vi "Heater PSU server.vi"() -> ()   [LabVIEW 2024]
doc: "Vi provides top level control program for TTICPX200 PSU used to drive the motor heater in the mechanical LTM"
uses:
  <userlib>/_OpenG.lib/comparison/comparison.llb/Boolean Changed__ogtk.vi
  <userlib>/_OpenG.lib/comparison/comparison.llb/DBL Changed__ogtk.vi
  <instrlib>/TTI CPX400/TTI CPX400.lvlib
  <userlib>/_OpenG.lib/comparison/comparison.llb/openg_comparison__ogtk.lvlib
panel:
  in  "Current Limit (600mA)":dbl=0.6 format="%.2g"
  out "Heater Monitor":waveform(dbl)[](array[waveform])
  in  "Heater PSU \nVISA name":refnum<visa-resource-name>="CPX400PSU"
  in  "Cadence":i64=100 min=1 max=1000
  out "Voltage":waveform(dbl)={"t0"=timestamp(3819958139.6161337 s since 1904-01-01), "dt"=1.0, "Y"=[-0.006], "attributes"=variant("NI_ChannelName"=variant(string "Heater_Voltage"))}
  out "I&V (Graph)":dynamicdata(graph)=[{"t0"=timestamp(3819958139.6161337 s since 1904-01-01), "dt"=1.0, "Y"=[-0.006], "attributes"=variant("NI_ChannelName"=variant(string "Heater_Voltage"))}, {"t0"=timestamp(3819958139.6161337 s since 1904-01-01), "dt"=1.0, "Y"=[-0.002], "attributes"=variant("NI_ChannelName"=variant(string "Heater_Current"))}]
  out "Current":waveform(dbl)={"t0"=timestamp(3819958139.6161337 s since 1904-01-01), "dt"=1.0, "Y"=[-0.002], "attributes"=variant("NI_ChannelName"=variant(string "Heater_Current"))}
  in  "stop":bool
  in  "Enable Output (T: Enable)":bool
  in  "Set Voltage":dbl=0.92 min=0.0 max=1.0 step=0.01 format="%.2f"
  in  "OCP Current (A)":dbl=1.0
  in  "OVP Voltage (V)":dbl=1.0
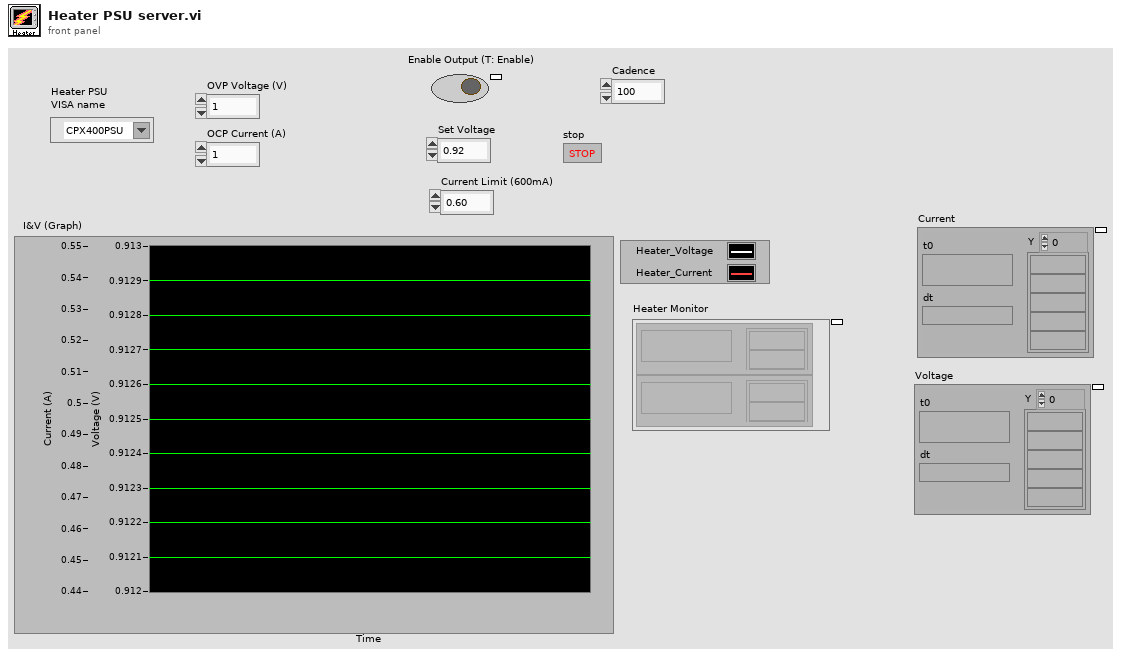
[diagram p1: front panel]
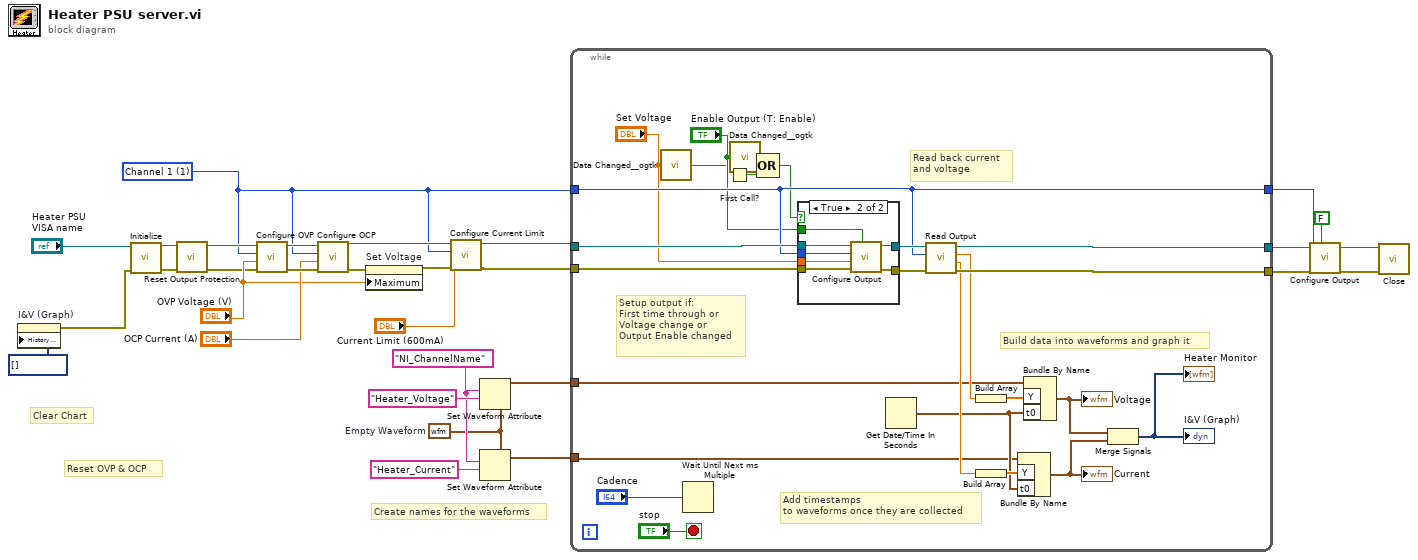
[diagram p0: block diagram]
diagram:
  w17 = "NI_ChannelName" ("name")
  w16 = waveform(dbl) {"t0"=timestamp(0 s since 1904-01-01), "dt"=1.0, "Y"=[]}  # Empty Waveform
  w2 = 1 items=["Channel 1"=1, "Channel 2"=2] ("Channel (1:Channel 1)")
  # "Clear Chart"
  # "Reset OVP & OCP"
  # "Create names for the waveforms"
  n1 = property on="I&V (Graph)" class="WFChart (strict)"("History Data"=dynamicdata[] []) -> (error out=w8:errorcluster)  [unwired: 2 in, 1 out]
  n2 = call <instrlib>:"Initialize.vi"("error in (no error)"=w8, "VISA resource name"="Heater PSU \nVISA name") -> ("error out"=w9:errorcluster, "VISA resource name out"=w11:refnum<visa-resource-name>)  [unwired: 8 in]
  n3 = call <instrlib>:"Reset Output Protection.vi"("error in (no error)"=w9, "VISA resource name"=w11) -> ("error out"=w10:errorcluster, "VISA resource name out"=w12:refnum<visa-resource-name>)  [unwired: 8 in]
  n4 = call <instrlib>:"Configure OVP.vi"("error in (no error)"=w10, "Voltage Limit (0.0 V)"="OVP Voltage (V)", "Channel (1: Channel 1)"=w2, "VISA resource name"=w12) -> ("error out"=w29:errorcluster, "VISA resource name out"=w28:refnum<visa-resource-name>)  [unwired: 6 in]
  n5 = call <instrlib>:"Configure OCP.vi"("error in (no error)"=w29, "Current Limit (0.0 A)"="OCP Current (A)", "Channel (1: Channel 1)"=w2, "VISA resource name"=w28) -> ("error out"=w14:errorcluster, "VISA resource name out"=w3:refnum<visa-resource-name>)  [unwired: 6 in]
  n6 = property on="Set Voltage" class="DigNum (strict)"(error in=w14, "Maximum"="OVP Voltage (V)") -> (error out=w5:errorcluster)  [unwired: 1 in, 1 out]
  n7 = call <instrlib>:"Configure Current Limit.vi"("error in (no error)"=w5, "Current Limit (0.0 A)"="Current Limit (600mA)", "Channel (1: Channel 1)"=w2, "VISA resource name"=w3) -> ("error out"=w6:errorcluster, "VISA resource name out"=w4:refnum<visa-resource-name>)  [unwired: 6 in]
  n8 = Set Waveform Attribute(5:"Heater_Voltage", 6:w17, 7:w16) -> (3:w20:waveform(dbl))  [unwired: 1 in, 2 out]
  n9 = Set Waveform Attribute(5:"Heater_Current", 6:w17, 7:w16) -> (3:w15:waveform(dbl))  [unwired: 1 in, 2 out]
  n10 = while {
    tunnel: w6 -> [w55]
    tunnel: w4 -> [w54]
    tunnel: w2 -> [w50]
    tunnel: [w50] -> w23
    tunnel: [w49] -> w22
    tunnel: [w48] -> w21
    tunnel: w20 -> [w38]
    tunnel: w15 -> [w37]
    stop <- "stop" stop-if-true
    # "Build data into waveforms and graph it"
    # "Read back current \nand voltage"
    # "Setup output if:\nFirst time through or\nVoltage change or\nOutput Enable changed"
    # "Add timestamps\nto waveforms once they are collected"
    n11 = call-poly <userlib>:"Data Changed__ogtk.vi"("DBL"="Set Voltage") -> ("Changed"=w34:bool)
    n12 = Wait Until Next ms Multiple(millisecond multiple="Cadence") -> ()  [unwired: 1 out]
    n13 = First Call?() -> (First Call?: T/F=w33:bool)
    n14 = call-poly <userlib>:"Data Changed__ogtk.vi"("Boolean"="Enable Output (T: Enable)") -> ("Changed"=w40:bool)
    n15 = Compound Arithmetic op=OR(w40, w34, w33) -> (w35:bool)
    n16 = case shown="True" w35 {
      tunnel: w55 -> [w56 w64]
      tunnel: w54 -> [w57 w63]
      tunnel: [w56 w62] -> w52
      tunnel: [w57 w61] -> w51
      tunnel: w50 -> [_ w60]
      tunnel: "Set Voltage" -> [_ w59]
      tunnel: "Enable Output (T: Enable)" -> [_ w58]
      frame False {
      }
      frame True {
        n17 = call <instrlib>:"Configure Output.vi"("Enable Output (T: Enable)"=w58, "error in (no error)"=w64, "Voltage Level (0.0 V)"=w59, "Channel (1: Channel 1)"=w60, "VISA resource name"=w63) -> ("error out"=w62:errorcluster, "VISA resource name out"=w61:refnum<visa-resource-name>)  [unwired: 5 in]
      }
    }
    n18 = Get Date/Time In Seconds() -> (seconds since 1Jan1904=w39:timestamp)
    n19 = call <instrlib>:"Read Output.vi"("error in (no error)"=w52, "Channel (1: Channel 1)"=w50, "VISA resource name"=w51) -> ("error out"=w48:errorcluster, "Actual Current Level (A)"=w47:dbl, "Actual Voltage Level (V)"=w45:dbl, "VISA resource name out"=w49:refnum<visa-resource-name>)  [unwired: 5 in]
    n20 = Build Array(w45) -> (w44:dbl[])
    n21 = Build Array(w47) -> (w46:dbl[])
    n22 = Bundle By Name(cluster=w37, "Y"=w46, "t0"=w39) -> (w42:waveform(dbl))
    "Current" <- w42
    n23 = Bundle By Name(cluster=w38, "Y"=w44, "t0"=w39) -> (w43:waveform(dbl))
    "Voltage" <- w43
    n24 = Merge Signals(w43, w42) -> (→"I&V (Graph)" →"Heater Monitor":dynamicdata)
  }
  n25 = call <instrlib>:"Configure Output.vi"("Enable Output (T: Enable)"=FALSE, "error in (no error)"=w21, "Channel (1: Channel 1)"=w23, "VISA resource name"=w22) -> ("error out"=w26:errorcluster, "VISA resource name out"=w25:refnum<visa-resource-name>)  [unwired: 6 in]
  n26 = call <instrlib>:"Close.vi"("error in (no error)"=w26, "VISA resource name"=w25) -> ()  [unwired: 9 in, 1 out]
